vi "target.vi"   [LabVIEW 2020]
uses:
  <vilib>/rvi/interface/RandomDataEmulation/niFpgaRandomDataHandleErrors.vi
  <vilib>/rvi/DataTransferAndStorage/Container/XNode/niFpgaContainer.xnode
  <vilib>/rvi/interface/RandomDataEmulation/nirviRandomDataFpgaReadWriteTemplate.vi
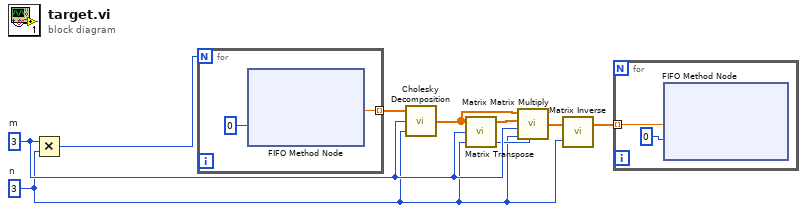
[diagram p0: block diagram]
diagram:
  w1 = 3  # n
  w7 = 3  # m
  n1 = Multiply(x=w7, y=w1) -> (x*y=w9:i32)
  n2 = for {
    N: w9 -> [_]
    tunnel: [w11] -> w8 mode=indexing
    n3 = xnode ("FIFO Method Node")("Timeout"=0) -> ("Element"=w11:sgl)  [unwired: 1 in, 2 out]
  }
  n4 = call <vilib>:"Cholesky Decomposition.vi"("n"=w1, "m"=w7, "A"=w8) -> ("L"=w6:sgl[])
  n5 = call <vilib>:"Matrix Transpose.vi"("n"=w1, "m"=w7, "A"=w6) -> ("n"=w4:i32, "B"=w5:sgl[])  [unwired: 1 out]
  n6 = call <vilib>:"Matrix Matrix Multiply.vi"("p"=w4, "n"=w1, "m"=w7, "B"=w5, "A"=w6) -> ("C"=w3:sgl[])  [unwired: 1 in]
  n7 = call <vilib>:"Matrix Inverse.vi"("n"=w1, "A"=w3) -> ("inv(A)"=w2:sgl[])  [unwired: 1 out]
  n8 = for {
    tunnel: w2 -> [w12] mode=indexing
    n9 = xnode ("FIFO Method Node")("Element"=w12, "Timeout"=0) -> ()  [unwired: 1 in, 2 out]
  }
